vi "HC-SR04 Read Distance.vi"(8 "error in (no error)":errorcluster, 10 "Temperature (deg C)":dbl=30.0, 11 "Trigger PIN":tag="C/DIO1") -> (0 "error out":errorcluster, 3 "Distance (m)":dbl)   [LabVIEW 2019]
doc: "Reads the distance in meters from the Parallax PING sensor located on the given pin.\n\nReturns -1 if the distance could not be read."
uses:
  <vilib>/myRIO/Instrument Drivers/Onboard IO/DIO/typedefs/DIO Reference.ctl
  <vilib>/myRIO/Common/Instrument Driver Framework/Utilities/typedefs/myRIO Generic Hardware Reference.ctl
  <vilib>/myRIO/Common/Instrument Driver Framework/Utilities/typedefs/Hardware Version Enum.ctl
  <vilib>/myRIO/Common/Instrument Driver Framework/Utilities/typedefs/myRIO v1.0 Reference.ctl
  <vilib>/myRIO/Common/Instrument Driver Framework/Utilities/typedefs/Generic FPGA Reference.ctl
  <vilib>/myRIO/Common/Instrument Driver Framework/myRIO v1.0/DIO/typedefs/DIO Channels List.ctl
  <vilib>/myRIO/Common/Instrument Driver Framework/myRIO v1.0/DIO/typedefs/DIO Channels Enum.ctl
  <vilib>/myRIO/Common/Instrument Driver Framework/myRIO v1.0/DIO/vis/myRIO v1.0 Close DIO.vi
  <vilib>/myRIO/Common/Instrument Driver Framework/myRIO v1.0/DIO/vis/myRIO v1.0 Unreserve DIO.vi
  <vilib>/myRIO/Common/Instrument Driver Framework/myRIO v1.0/DIO/vis/myRIO v1.0 Build MUX Configuration DIO.vi
  <vilib>/myRIO/Common/Instrument Driver Framework/myRIO v1.0/Resource Manager/vis/myRIO v1.0 Unreserve Channel List.vi
  <vilib>/myRIO/Common/Instrument Driver Framework/myRIO v1.0/Resource Manager/vis/myRIO v1.0 Create Configuration List.vi
  <vilib>/myRIO/Common/Instrument Driver Framework/myRIO v1.0/Resource Manager/vis/myRIO v1.0 Unreserve Channel.vi
  <vilib>/myRIO/Common/Instrument Driver Framework/myRIO v1.0/Resource Manager/vis/myRIO v1.0 Build Mutex Name.vi
  <vilib>/Utility/error.llb/Error Cluster From Error Code.vi
  <vilib>/myRIO/Common/Instrument Driver Framework/myRIO v1.0/DIO/vis/myRIO v1.0 Write DIO.vi
  <vilib>/myRIO/Common/Instrument Driver Framework/myRIO v1.0/DIO/vis/myRIO v1.0 Read DIO.vi
  <vilib>/myRIO/Common/Instrument Driver Framework/myRIO v1.0/DIO/vis/myRIO v1.0 Shutdown DIO.vi
  <vilib>/myRIO/Common/Instrument Driver Framework/myRIO v1.0/Resource Manager/vis/myRIO v1.0 Configure IO.vi
  <vilib>/myRIO/Common/Instrument Driver Framework/Utilities/vis/Configuration Manager.vi
  <vilib>/myRIO/Common/Instrument Driver Framework/Utilities/vis/IO Manager.vi
  <vilib>/myRIO/Common/Instrument Driver Framework/myRIO v1.0/myRIO v1.0 Close.vi
  <vilib>/myRIO/Instrument Drivers/Onboard IO/DIO/DIO.lvlib
panel:
  out "error out 2":errorcluster
  in  "stop":bool
  in  "Echo PIN":tag="C/DIO1"
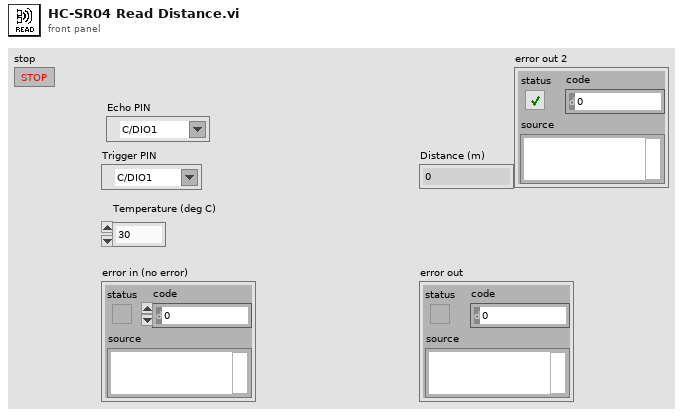
[diagram p1: front panel]
types:
  T1 = enum16{"Initialize", "Trigger pulse", "Wait for rising edge", "Wait for falling edge", "Calculate distance", "Stop"}
  T2 = typedef "DIO.lvlib/DIO Reference.ctl" = cluster{"myRIO Reference":T3, "DIO Channels List":T7}
  T3 = typedef "myRIO Generic Hardware Reference.ctl" = cluster{"myRIO Model":T4, "myRIO Hardware Reference":T5}
  T4 = typedef "Hardware Version Enum.ctl" = enum16{"Unknown", "myRIO-1900", "myRIO-1950", "roboRIO", "NI ELVIS RIO CM", "ELVIS III"}
  T5 = typedef "myRIO v1.0 Reference.ctl" = cluster{"Generic FPGA Reference":T6, "Allow multiple opens":bool}
  T6 = typedef "Generic FPGA Reference.ctl" = refnum<k20>
  T7 = typedef "DIO Channels List.ctl" = T8[]
  T8 = typedef "DIO Channels Enum.ctl" = enum16{"Not Connected", "C/DIO0", "C/DIO1", "C/DIO2", "C/DIO3", "C/DIO4", "C/DIO5", "C/DIO6", "C/DIO7", "A/DIO0", "A/DIO1", "A/DIO2", "A/DIO3", "A/DIO4", "A/DIO5", "A/DIO6", "A/DIO7", "A/DIO8", "A/DIO9", "A/DIO10", "A/DIO11", "A/DIO12", "A/DIO13", "A/DIO14", "A/DIO15", "A/DIO16", "A/DIO17", "A/DIO18", "A/DIO19", "B/DIO0", "B/DIO1", "B/DIO2", "B/DIO3", "B/DIO4", "B/DIO5", "B/DIO6", "B/DIO7", "B/DIO8", "B/DIO9", "B/DIO10", "B/DIO11", "B/DIO12", "B/DIO13", "B/DIO14", "B/DIO15", "B/DIO16", "B/DIO17", "B/DIO18", "B/DIO19", "LED0", "LED1", "LED2", "LED3", "Button0", "DIO/DIO0", "DIO/DIO1", "DIO/DIO2", "DIO/DIO3", "DIO/DIO4", "DIO/DIO5", "DIO/DIO6", "DIO/DIO7", "DIO/DIO8", "DIO/DIO9", "SPI/CS0", "SPI/CS1", "SPI/CS2", "SPI/CS3", "LED RADIO (Green)", "LED RADIO (Red)", "LED COMM (Green)", "LED COMM (Red)", "LED MODE (Green)", "LED MODE (Red)"}
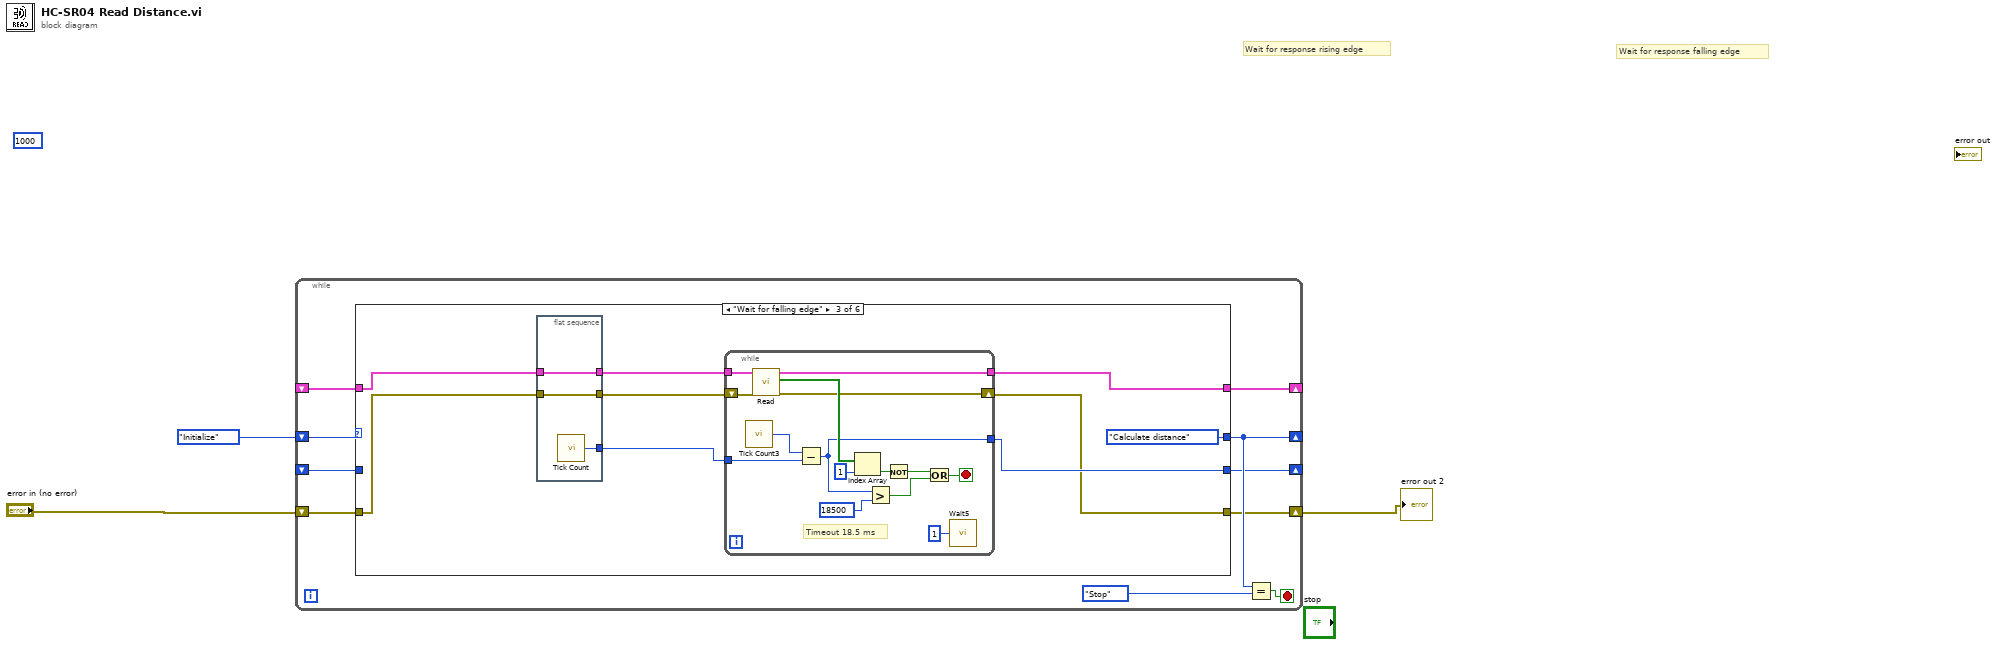
[diagram p0: block diagram]
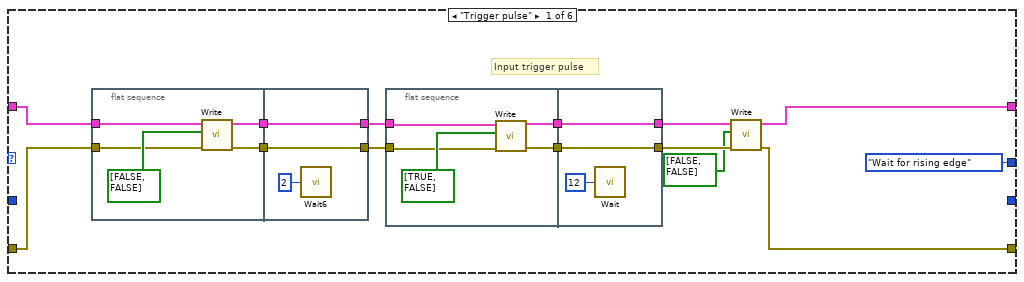
[diagram p2: hidden frame]
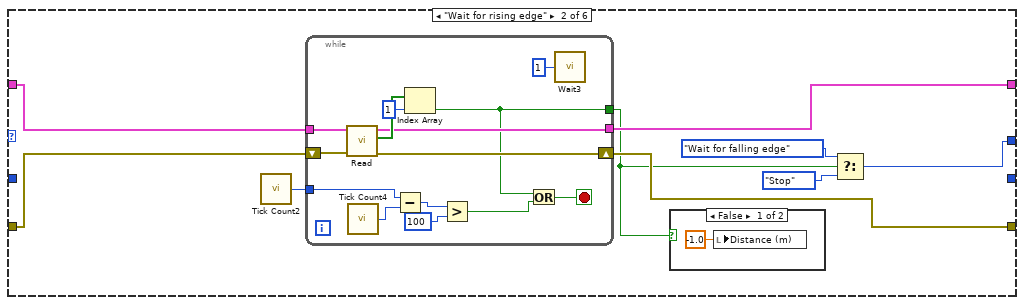
[diagram p3: hidden frame]
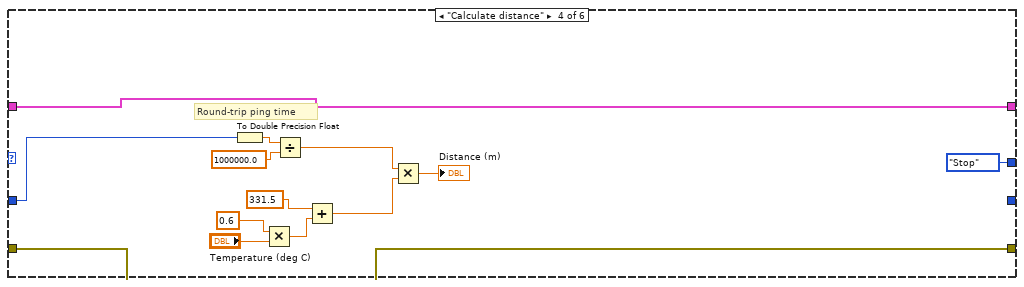
[diagram p5: hidden frame]
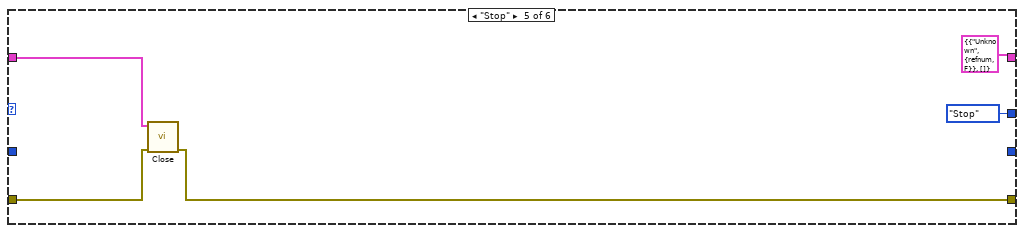
[diagram p6: hidden frame]
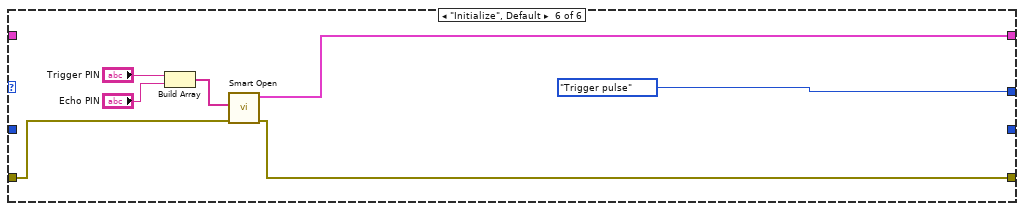
[diagram p7: hidden frame]
diagram:
  (unwired) i64 1000 ("Period")
  # "Wait for response falling edge"
  # "Wait for response rising edge"
  n1 = while {
    shift-right: [w12] -> _
    shift-left: T1."Initialize" -> [w11]
    shift-right: [w6] -> w2
    shift-left: "error in (no error)" -> [w9]
    shift-right: [w8] -> _
    shift-left: _ -> [w7]
    shift-right: [w5] -> _
    shift-left: _ -> [w4]
    stop <- w13 stop-if-true
    n2 = case shown="\"Wait for falling edge\"" w11 {
      tunnel: [T1."Wait for rising edge" w48 T1."Calculate distance" ("y") T1."Stop" ("y") T1."Stop" ("y") T1."Trigger pulse"] -> w12
      tunnel: w9 -> [w18 w51 w72 w95 w111 w117]
      tunnel: [w16 w47 w71 w98 T2 {"myRIO Reference"={"myRIO Model"=enum."Unknown", "myRIO Hardware Reference"={"Generic FPGA Reference"=refnum, "Allow multiple opens"=FALSE}}, "DIO Channels List"=[]} ("DIO Ref Out") w116] -> w8
      tunnel: w7 -> [w17 w52 w73 w98 w110 _]
      tunnel: [w15 w46 w68 w95 w109 w115] -> w6
      tunnel: [_ _ w70 _ _ _] -> w5
      tunnel: w4 -> [_ _ _ w97 _ _]
      frame "Trigger pulse" {
        # "Input trigger pulse"
        n3 = flat-sequence {
          tunnel: [w31] -> w25
          tunnel: [w30] -> w24
          tunnel: w18 -> [w29]
          tunnel: w17 -> [w28]
          tunnel: [w34] -> w22
          tunnel: [w33] -> w23
          tunnel: w25 -> [w34]
          tunnel: w24 -> [w33]
          frame #0 {
            n4 = call <vilib>:"Write.vi"("error in (no error)"=w29, "Values"=bool[] [FALSE, FALSE], "DIO Ref In"=w28) -> ("error out"=w30:errorcluster, "DIO Ref Out"=w31:T2)  [unwired: 6 in]
          }
          frame #1 {
            n5 = call "Wait6"("Count(uSec)"=u32 2) -> ()  [unwired: 1 out]
          }
        }
        n6 = flat-sequence {
          tunnel: [w39] -> w27
          tunnel: [w38] -> w26
          tunnel: w23 -> [w37]
          tunnel: w22 -> [w36]
          tunnel: [w42] -> w19
          tunnel: [w41] -> w21
          tunnel: w27 -> [w42]
          tunnel: w26 -> [w41]
          frame #0 {
            n7 = call <vilib>:"Write.vi"("error in (no error)"=w37, "Values"=bool[] [TRUE, FALSE], "DIO Ref In"=w36) -> ("error out"=w38:errorcluster, "DIO Ref Out"=w39:T2)  [unwired: 6 in]
          }
          frame #1 {
            n8 = call "Wait"("Count(uSec)"=u32 12) -> ()  [unwired: 1 out]
          }
        }
        n9 = call <vilib>:"Write.vi"("error in (no error)"=w21, "Values"=bool[] [FALSE, FALSE], "DIO Ref In"=w19) -> ("error out"=w15:errorcluster, "DIO Ref Out"=w16:T2)  [unwired: 6 in]
      }
      frame "Wait for rising edge" {
        n10 = call "Tick Count2"() -> ("Tick Count(uSec)"=w44:u32)
        n11 = while {
          tunnel: [w65] -> w47
          shift-right: [w63] -> w46
          shift-left: w51 -> [w64]
          tunnel: w44 -> [w60]
          tunnel: w52 -> [w62]
          tunnel: [w55] -> w45
          stop <- w57 stop-if-true
          n12 = call <vilib>:"Read.vi"("error in (no error)"=w64, "DIO Ref In"=w62) -> ("error out"=w63:errorcluster, "Values"=w66:bool[], "DIO Ref Out"=w65:T2)  [unwired: 7 in]
          n13 = call "Tick Count4"() -> ("Tick Count(uSec)"=w61:u32)
          n14 = Subtract(x=w60, y=w61) -> (x-y=w59:u32)
          n15 = Index Array(array=w66, index=1) -> (element=w55:bool)
          n16 = Greater?(x=w59, y=u32 100) -> (0:w56:bool)
          n17 = Or(x=w55, y=w56) -> (x .or. y?=w57:bool)
          n18 = call "Wait3"("Count(uSec)"=u32 1) -> ()  [unwired: 1 out]
        }
        n19 = case shown="False" w45 {
          frame False {
            n20 = local write "Distance (m)"(-1.0 ("Distance (m)")) -> ()
          }
          frame True {
          }
        }
        n21 = Select(t=T1."Wait for falling edge", s=w45, f=T1."Stop" ("y")) -> (s? t:f=w48:T1)
      }
      frame "Wait for falling edge" {
        n22 = flat-sequence {
          tunnel: w73 -> [w94]
          tunnel: w72 -> [w92]
          tunnel: [w94] -> w76
          tunnel: [w93] -> w75
          tunnel: [w92] -> w74
          frame #0 {
            n23 = call "Tick Count"() -> ("Tick Count(uSec)"=w93:u32)
          }
        }
        n24 = while {
          tunnel: w76 -> [w90]
          tunnel: w75 -> [w87]
          shift-right: [w81] -> w68
          shift-left: w74 -> [w82]
          tunnel: [w79] -> w71
          tunnel: [w78] -> w70
          stop <- w86 stop-if-true
          # "Timeout 18.5 ms"
          n25 = call "Tick Count3"() -> ("Tick Count(uSec)"=w80:u32)
          n26 = call <vilib>:"Read.vi"("error in (no error)"=w82, "DIO Ref In"=w90) -> ("error out"=w81:errorcluster, "Values"=w89:bool[], "DIO Ref Out"=w79:T2)  [unwired: 7 in]
          n27 = Subtract(x=w80, y=w87) -> (x-y=w78:u32)
          n28 = Index Array(array=w89, index=1) -> (element=w88:bool)
          n29 = Greater?(x=w78, y=u32 18500) -> (0:w84:bool)
          n30 = Not(x=w88) -> (.not. x?=w85:bool)
          n31 = Or(x=w85, y=w84) -> (x .or. y?=w86:bool)
          n32 = call "Wait5"("Count(uSec)"=u32 1) -> ()  [unwired: 1 out]
        }
      }
      frame "Calculate distance" {
        # "Round-trip ping time"
        n33 = To Double Precision Float(number=w97) -> (double precision float=w103:dbl)
        n34 = Multiply(x=0.6, y="Temperature (deg C)") -> (x*y=w101:dbl)
        n35 = Divide(x=w103, y=1000000.0) -> (x/y=w105:dbl)
        n36 = Add(x=331.5, y=w101) -> (x+y=w106:dbl)
        n37 = Multiply(x=w105, y=w106) -> (x*y=→"Distance (m)":dbl)
      }
      frame "Stop" {
        n38 = call <vilib>:"Close.vi"("error in (no error)"=w111, "DIO Ref In"=w110) -> ("error out"=w109:errorcluster)  [unwired: 9 in]
      }
      frame "Initialize", Default {
        n39 = Build Array("Trigger PIN", "Echo PIN") -> (w119:tag[])
        n40 = call <vilib>:"Smart Open.vi"("error in (no error)"=w117, "Channel Names"=w119) -> ("error out"=w115:errorcluster, "DIO Ref Out"=w116:T2)  [unwired: 8 in]
      }
    }
    n41 = Equal?(x=w12, y=T1."Stop") -> (x = y?=w13:bool)
  }
  "error out 2" <- w2
